vi "BK Precision 5490C Series Acquire Triggered Multiple.vi"() -> ()   [LabVIEW 2018]
doc: "This example shows how to configure a measurement, set up trigger and sampling count, and trigger and fetch measurement."
uses:
  <instrlib>/BK Precision 5490C Series/BK Precision 5490C Series.lvlib
panel:
  in  "Measurement Function (0: Voltage DC)":i32(ring) items=["Voltage DC", "Voltage DC Ratio", "Voltage AC", "Current DC", "Current AC", "Resistance 2-Wire", "Resistance 4-Wire", "Frequency", "Period", "Capacitance", "Continuity", "Diode", "Temperature"]
  in  "Sample Count (1)":i32=1 format="%#.6g"
  in  "Trigger Count (1)":i32=1 format="%#.6g"
  in  "VISA resource name":refnum<visa-resource-name>
  out "Waveform Chart":dbl[](graph)
  # "(c) 2020 B&K Precision Corporation.  ALL RIGHTS RESERVED."
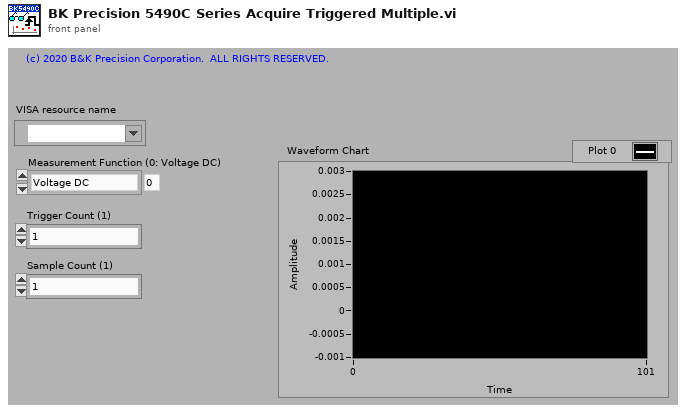
[diagram p1: front panel]
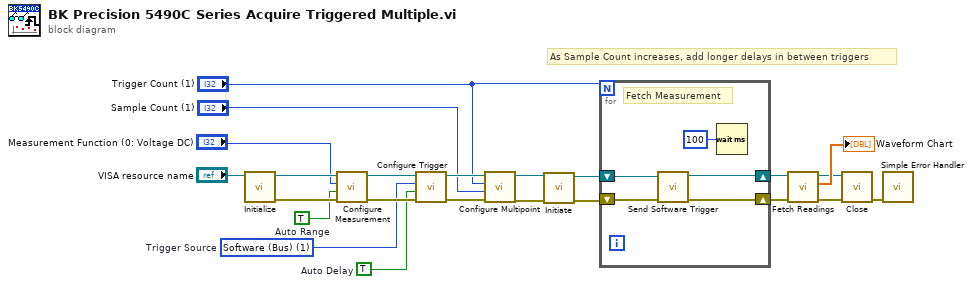
[diagram p0: block diagram]
diagram:
  w10 = 1 items=["Immediate", "Software (Bus)", "External"]  # Trigger Source
  w15 = TRUE  # Auto Range
  w16 = TRUE  # Auto Delay
  # "As Sample Count increases, add longer delays in between triggers"
  n1 = call <instrlib>:"Initialize.vi"("VISA resource name"="VISA resource name") -> ("error out"=w22:errorcluster, "VISA resource name out"=w23:refnum<visa-resource-name>)  [unwired: 4 in, 5 out]
  n2 = call <instrlib>:"Configure Measurement.vi"("error in (no error)"=w22, "Auto Range (T: Enable)"=w15, "Measurement Function (0: Voltage DC)"="Measurement Function (0: Voltage DC)", "VISA resource name"=w23) -> ("error out"=w20:errorcluster, "VISA resource name out"=w21:refnum<visa-resource-name>)  [unwired: 1 in, 5 out]
  n3 = call <instrlib>:"Configure Trigger.vi"("error in (no error)"=w20, "Auto Delay (T:Enable)"=w16, "Trigger Source (0: Immediate)"=w10, "VISA resource name"=w21) -> ("error out"=w18:errorcluster, "VISA resource name out"=w19:refnum<visa-resource-name>)  [unwired: 1 in, 5 out]
  n4 = call <instrlib>:"Configure Multipoint.vi"("error in (no error)"=w18, "Sample Count (1)"="Sample Count (1)", "Trigger Count (1)"="Trigger Count (1)", "VISA resource name"=w19) -> ("error out"=w13:errorcluster, "VISA resource name out"=w14:refnum<visa-resource-name>)  [unwired: 6 out]
  n5 = call <instrlib>:"Initiate.vi"("error in (no error)"=w13, "VISA resource name"=w14) -> ("error out"=w12:errorcluster, "VISA resource name out"=w11:refnum<visa-resource-name>)  [unwired: 8 out]
  n6 = for {
    N: "Trigger Count (1)" -> [_]
    shift-right: [w25] -> w5
    shift-left: w12 -> [w27]
    shift-right: [w26] -> w4
    shift-left: w11 -> [w28]
    # "Fetch Measurement"
    n7 = call <instrlib>:"Send Software Trigger.vi"("error in (no error)"=w27, "VISA resource name"=w28) -> ("error out"=w25:errorcluster, "VISA resource name out"=w26:refnum<visa-resource-name>)  [unwired: 8 out]
    n8 = Wait (ms)(milliseconds to wait=u32 100) -> ()  [unwired: 1 out]
  }
  n9 = call <instrlib>:"Fetch Readings.vi"("error in (no error)"=w5, "VISA resource name"=w4) -> ("error out"=w7:errorcluster, "Measurements"=→"Waveform Chart":dbl[], "VISA resource name out"=w6:refnum<visa-resource-name>)  [unwired: 2 in, 5 out]
  n10 = call <instrlib>:"Close.vi"("error in (no error)"=w7, "VISA resource name"=w6) -> ("error out"=w17:errorcluster)  [unwired: 9 out]
  n11 = call <vilib>:"Simple Error Handler.vi"("error in (no error)"=w17) -> ()  [unwired: 1 in, 8 out]
